vi "DAC Save Results.vi"(8 "error in":errorcluster, 9 "Log Details?":bool, 10 "tdms file":refnum<k34>, 11 "DAC Shunt dU in":refnum<class "DAC Shunt dU.lvclass">) -> (0 "error out":errorcluster)   [LabVIEW 2019, in "DAC.lvlib" / "DAC Shunt dU.lvclass"]
uses:
  DAC Shunt dU.lvclass
  C:/Users/krio/Documents/LV_Projects/TestStand/App/DAC/DAC.lvclass
  DAC.lvclass/DAC.ctl
  DAC Shunt dU.lvclass/DAC Shunt dU.ctl
  DAC.lvclass
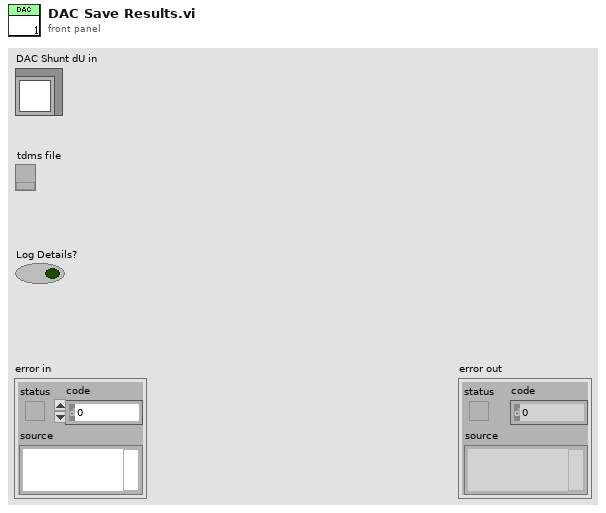
[diagram p1: front panel]
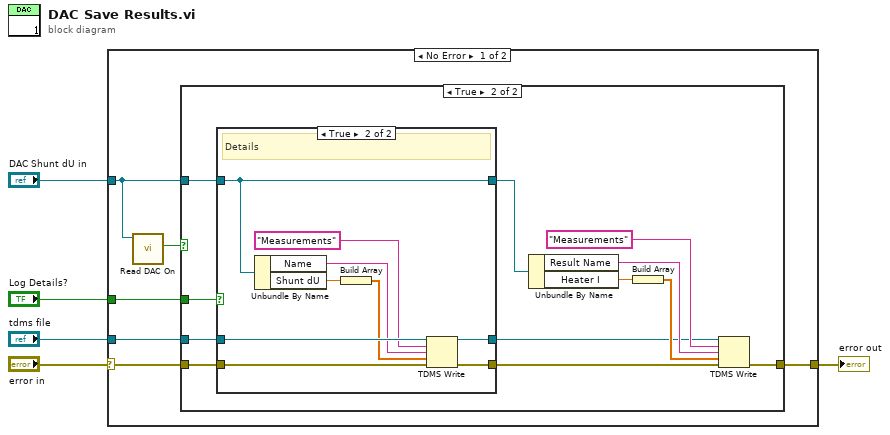
[diagram p0: block diagram]
diagram:
  n1 = case shown="No Error" "error in" {
    selector: "error in" -> [w8 w37]
    tunnel: "DAC Shunt dU in" -> [w11 _]
    tunnel: "tdms file" -> [w9 _]
    tunnel: [w7 w37] -> w2
    tunnel: "Log Details?" -> [w6 _]
    frame No Error {
      n2 = call "Read DAC On.vi"("DAC in"=w11) -> ("DAC On"=w10:bool)  [unwired: 8 in, 2 out]
      n3 = case shown="True" w10 {
        tunnel: w11 -> [_ w22]
        tunnel: w9 -> [_ w24]
        tunnel: w8 -> [w12 w23]
        tunnel: [w12 w13] -> w7
        tunnel: w6 -> [_ w21]
        frame False {
        }
        frame True {
          n4 = case shown="True" w21 {
            tunnel: w24 -> [w26 w36]
            tunnel: w23 -> [w27 w32]
            tunnel: w22 -> [w25 w29]
            tunnel: [w27 w31] -> w15
            tunnel: [w26 w30] -> w16
            tunnel: [w25 w29] -> w14
            frame False {
            }
            frame True {
              # "Details"
              n5 = Unbundle By Name(w29) -> ("Name"=w34:string, "Shunt dU"=w35:dbl)
              n6 = Build Array(w35) -> (w28:dbl[])
              n7 = TDMS Write(0:w36, 5:"Measurements" ("group name in (Untitled)"), 7:w34, 9:w28, 11:w32) -> (4:w30:refnum<k34>, 15:w31:errorcluster)  [unwired: 1 in, 2 out]
            }
          }
          n8 = Unbundle By Name(w14) -> ("Result Name"=w18:string, "Heater I"=w20:dbl)
          n9 = Build Array(w20) -> (w19:dbl[])
          n10 = TDMS Write(0:w16, 5:"Measurements" ("group name in (Untitled)"), 7:w18, 9:w19, 11:w15) -> (15:w13:errorcluster)  [unwired: 1 in, 3 out]
        }
      }
    }
    frame Error {
    }
  }
  "error out" <- w2
